vi "Mode PtByPt.vi"(2 "initialize":bool, 3 "sample length":i32=100, 4 "intervals":i32=1, 5 "x":dbl format="%0.2f") -> (0 "error":i32, 1 "mode":dbl format="%0.2f")   [LabVIEW 2020, in "NI_PtbyPt.lvlib"]
doc: "Finds the <B>mode</B> of the set of input data points specified by <B>sample length</B> by computing the histogram of the input values and selecting the largest bin. The <B>mode</B> is the center value of the bin with the largest count."
uses:
  <vilib>/ptbypt/NI_PtbyPt.lvlib
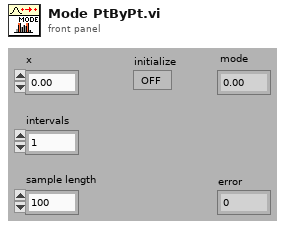
[diagram p1: front panel]
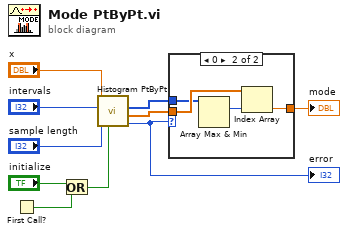
[diagram p0: block diagram]
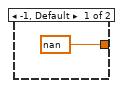
[diagram p2: hidden frame]
diagram:
  n1 = First Call?() -> (First Call?: T/F=w2:bool)
  n2 = Or(x="initialize", y=w2) -> (x .or. y?=w3:bool)
  n3 = call <vilib>:"Histogram PtByPt.vi"("initialize"=w3, "sample length"="sample length", "intervals"="intervals", "x"="x") -> ("error"=w1:i32, "X Values"=w9:dbl[], "Histogram: h(x)"=w8:i32[])  [unwired: 4 in, 1 out]
  "error" <- w1
  n4 = case shown="0" w1 {
    tunnel: w9 -> [_ w14]
    tunnel: w8 -> [_ w13]
    tunnel: [nan w12] -> w7
    frame -1, Default {
    }
    frame 0 {
      n5 = Array Max & Min(array=w13) -> (max index (indices)=w15:i32)  [unwired: 3 out]
      n6 = Index Array(array=w14, index=w15) -> (element=w12:dbl)
    }
  }
  "mode" <- w7
